vi "Client.vi"() -> ()   [LabVIEW 2015]
panel:
  out "Data Recv":string
  in  "Data Send":string="Test data client"
  in  "IPv6 Port":dbl=1050.0
  in  "IPv6 Address":string="2001:0DB8:AC10:FE01:0000:0000:0000:0000"
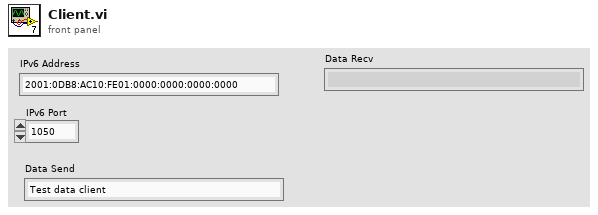
[diagram p1: front panel]
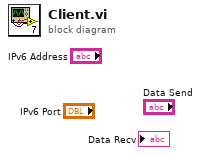
[diagram p0: block diagram]
diagram:
